vi "Drive and Climb SS Outputs 2017.vi"(11 "Drive Actuator In":T3) -> (0 "error out":T1)   [LabVIEW 2016]
uses:
  Drive Actuator Out 2017.ctl
  Drive and Climb Errors.ctl
  <vilib>/Rock Robotics/WPI/DriverStation/WPI_DriverStationRobotMode2.ctl
  Drive and Climb Logging Values.vi
  Global Variables/Refnum Names.vi
  <vilib>/Rock Robotics/WPI/Solenoid/WPI_SolenoidSetEnum.vi
  Global Variables/Robot Status.vi
  Robot Global Data.vi
  Global Variables/Sensor Data.vi
panel:
  out "Right Drive Commanded Speed":dbl
  out "Right Sensor Velocity":dbl
  out "Left Drive Commanded Speed":dbl
  out "Left Sensor Velocity":dbl
  out "Right Drive Motors":T2(graph)
  out "Left Drive Motors":T2(graph)
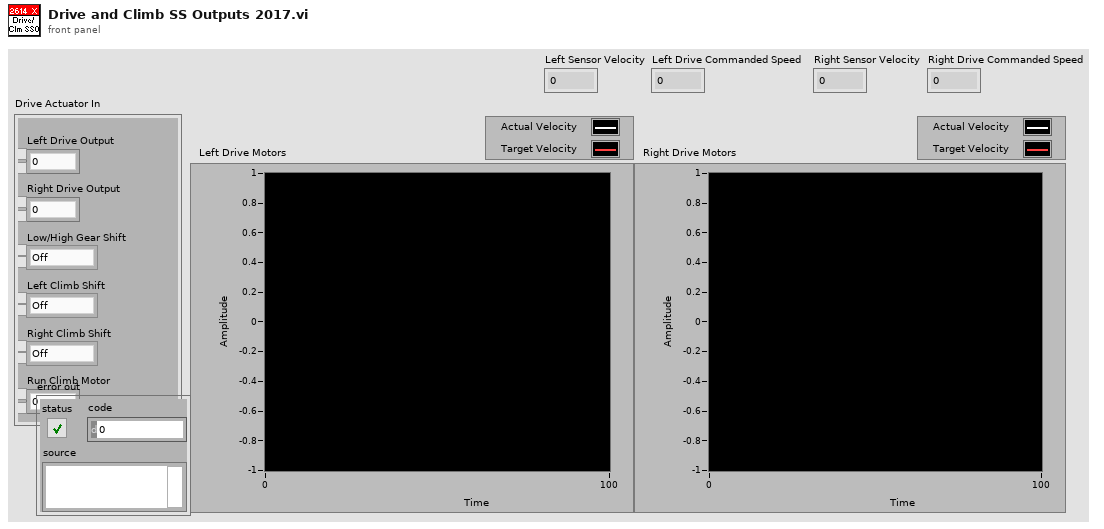
[diagram p1: front panel]
types:
  T1 = typedef "Drive and Climb Errors.ctl" = errorcluster
  T2 = cluster{"Encoder Velocity":dbl, "Left Drive Output":dbl}
  T3 = typedef "Drive Actuator Out 2017.ctl" = cluster{"Left Drive Output":dbl, "Right Drive Output":dbl, "Low/High Gear Shift":enum16{"Off", "On", "Forward", "Reverse"}, "Left Climb Shift":enum16{"Off", "On", "Forward", "Reverse"}, "Right Climb Shift":enum16{"Off", "On", "Forward", "Reverse"}, "Run Climb Motor":dbl}
  T4 = typedef "WPI_DriverStationRobotMode2.ctl" = enum16{"Autonomous Disabled", "Autonomous Enabled", "Teleop Disabled", "Teleop Enabled", "Disconnected", "Finish", "Test Disabled", "Test Enabled", "Emergency Stopped"}
  T5 = typedef "WPI_SolenoidDevRef.ctl" = cluster{"DevStatus":errorcluster, "Pneumatics Control Module":u8, "Forward Solenoid Channel":T6, "Reverse Solenoid Channel":T6}
  T6 = typedef "WPI_SolenoidChannel.ctl" = enum8{"Solenoid 0", "Solenoid 1", "Solenoid 2", "Solenoid 3", "Solenoid 4", "Solenoid 5", "Solenoid 6", "Solenoid 7", "Invalid"}
  T7 = typedef "WPI_MotorControlDeviceRef.ctl" = cluster{"DeviceStatus":errorcluster, "Type":T8, "PWM":cluster{"PWM Channel":T9, "DeadBand":T10}, "CAN":cluster{"Device Number":u8, "SetOutput VI Ref":variant, "GetOutput VI Ref":variant, "Enable VI Ref":variant, "Disable VI Ref":variant, "Data":variant}, "Invert":bool}
  T8 = typedef "WPI_MotorControlType.ctl" = enum16{"PWM", "CAN"}
  T9 = typedef "FPGA_DIOPWMChannel.ctl" = enum8{"PWM 0", "PWM 1", "PWM 2", "PWM 3", "PWM 4", "PWM 5", "PWM 6", "PWM 7", "PWM 8", "PWM 9", "PWM MXP 0", "PWM MXP 1", "PWM MXP 2", "PWM MXP 3", "PWM MXP 4", "PWM MXP 5", "PWM MXP 6", "PWM MXP 7", "PWM MXP 8", "PWM MXP 9", "Invalid"}
  T10 = typedef "WPI_PWMDeadband.ctl" = cluster{"Name":string, "maxPositivePwm":i32, "minPositivePwm":i32, "centerPwm":i32, "maxNegativePwm":i32, "minNegativePwm":i32, "angularRange":u16}
  T11 = typedef "WPI_CANTalonSRX_GlobalStatus.ctl" = cluster{"Applied Throttle":dbl, "Module Enabled":bool, "CAN Error":errorcluster, "Closed Loop Error":dbl, "Forward Limit Switch Closed":bool, "Reverse Limit Switch Closed":bool, "Sensor Position":dbl, "Sensor Velocity":dbl, "Current":dbl, "Sticky Fault - Over Temp":bool, "Sticky Fault - Under Voltage":bool, "Sticky Fault - Forward Limit":bool, "Sticky Fault - Reverse Limit":bool, "Sticky Fault - Forward Soft Limit":bool, "Sticky Fault - Reverse Soft Limit":bool, "Brake is Enabled":bool, "Encoder Position":dbl, "Encoder Velocity":dbl, "Encoder Index Count":dbl, "Encoder A Pin State":bool, "Encoder B Pin State":bool, "Encoder Index Pin State":bool, "Analog In":dbl, "Analog In Velocity":dbl, "Temperature (C)":dbl, "Battery Voltage":dbl, "Control 5 Is Supported":bool, "Current Profile Slot Select":dbl, "Pos Div 8":bool, "Vel Div 4":bool, "Pulse Width Position":i32, "Pulse Width Velocity":i32, "Pulse Width Rise To Rise (us)":i32, "Pulse Width Rise To Fall (us)":i32, "Mot Prof Active Is Under Run":bool, "Mot Prof Active Has Under Run":bool, "Mot Prof Active Is Last":bool, "Mot Prof Active Velocity Only":bool, "Mot Prof Active Is Valid":bool, "Mot Prof Buffer Is Full":bool, "Mot Prof Active Profile Slot Select":i32, "Mot Prof NextID":i32, "Mot Prof Count":i32, "Mot Prof Active Velocity":dbl, "Mot Prof Active Position":dbl, "Mot Prof Output Enable":i32, "UsageFrame":u32, "Motion Magic Active Trajectory":cluster{"Velocity":dbl, "Position":dbl}}
  T12 = cluster{"Sensor Velocity":dbl, "Right Drive Output":dbl}
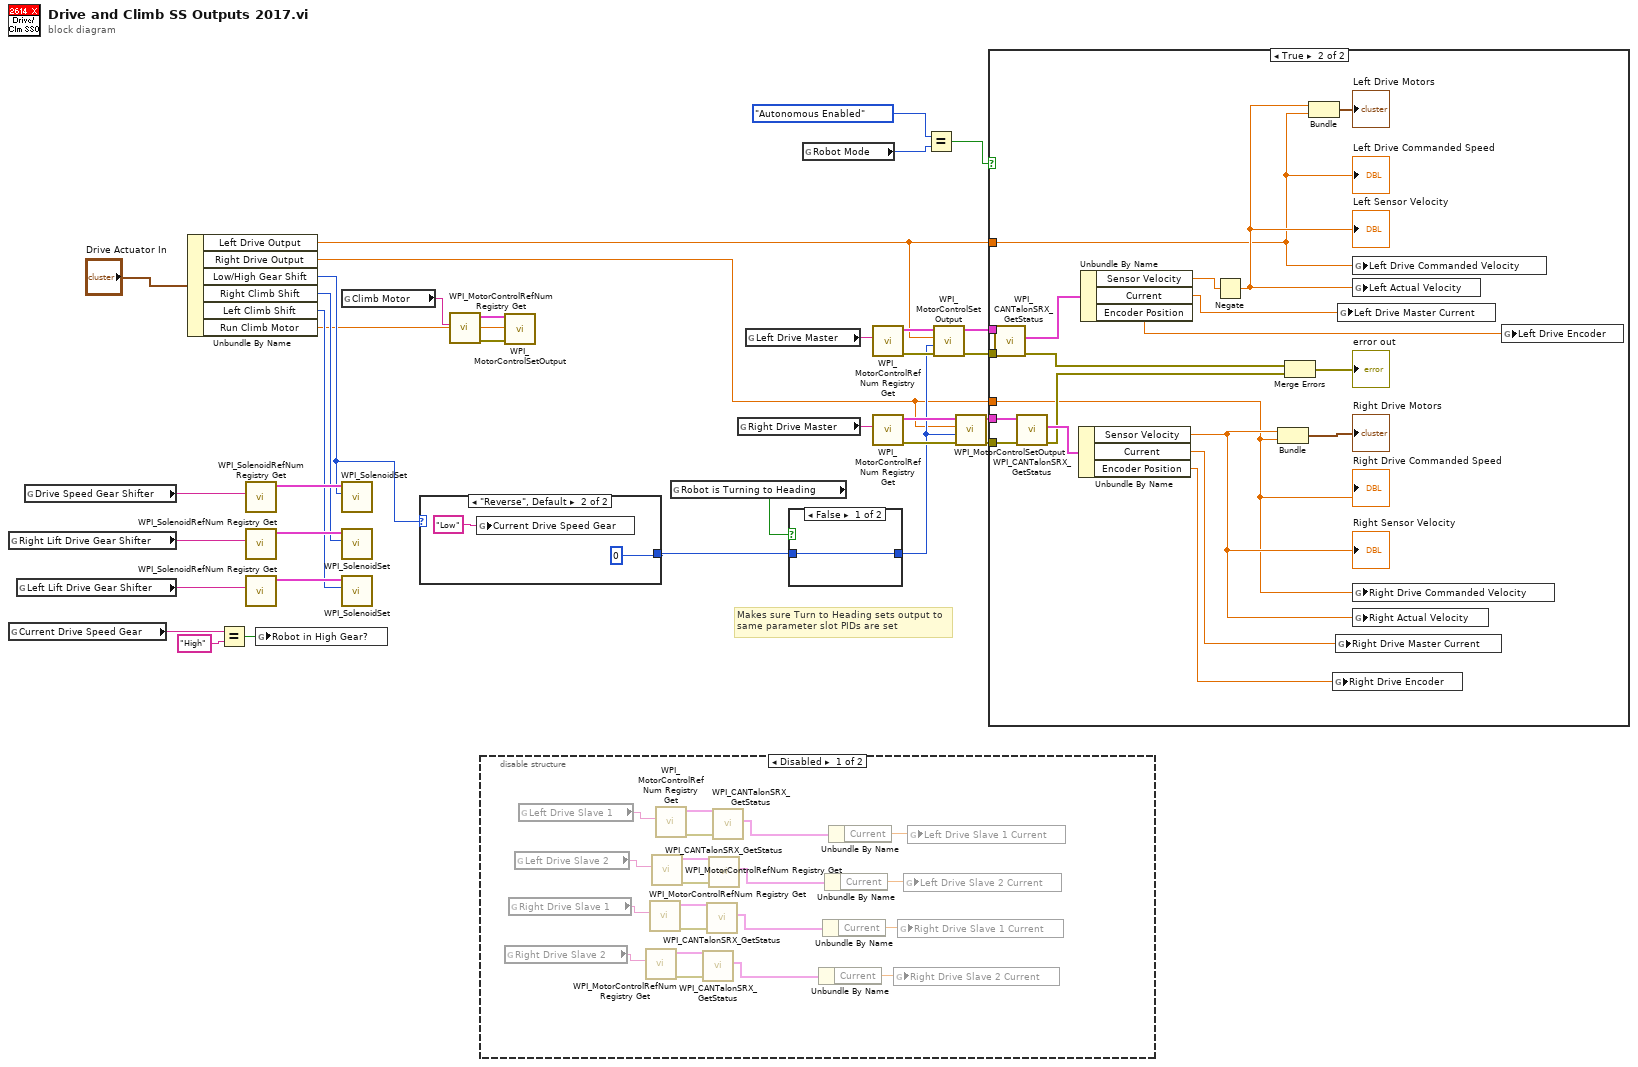
[diagram p0: block diagram]
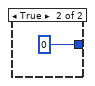
[diagram p4: hidden frame]
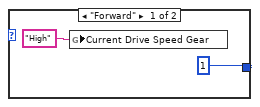
[diagram p5: hidden frame]
diagram:
  # "Makes sure Turn to Heading sets output to same parameter slot PIDs are set"
  n1 = global read "Refnum Names.vi" "Right Lift Drive Gear Shifter"() -> (w22:string)
  n2 = global read "Drive and Climb Logging Values.vi" "Current Drive Speed Gear"() -> (w12:string)
  n3 = global read "Refnum Names.vi" "Left Lift Drive Gear Shifter"() -> (w19:string)
  n4 = global read "Refnum Names.vi" "Drive Speed Gear Shifter"() -> (w30:string)
  n5 = Unbundle By Name("Drive Actuator In") -> ("Left Drive Output"=w8:dbl, "Right Drive Output"=w9:dbl, "Low/High Gear Shift"=w10:enum16{"Off", "On", "Forward", "Reverse"}, "Right Climb Shift"=w17:enum16{"Off", "On", "Forward", "Reverse"}, "Left Climb Shift"=w16:enum16{"Off", "On", "Forward", "Reverse"}, "Run Climb Motor"=w4:dbl)
  n6 = Equal?(x=w12, y="High") -> (x = y?=w15:bool)
  n7 = call <vilib>:"WPI_SolenoidRefNum Registry Get.vi"("refnum name"=w30) -> ("SolenoidDevRef"=w29:T5)  [unwired: 9 in, 1 out]
  n8 = call <vilib>:"WPI_SolenoidRefNum Registry Get.vi"("refnum name"=w22) -> ("SolenoidDevRef"=w21:T5)  [unwired: 9 in, 1 out]
  n9 = call <vilib>:"WPI_SolenoidRefNum Registry Get.vi"("refnum name"=w19) -> ("SolenoidDevRef"=w20:T5)  [unwired: 9 in, 1 out]
  n10 = global write "Robot Status.vi" "Robot in High Gear?"(w15) -> ()
  n11 = global read "Refnum Names.vi" "Climb Motor"() -> (w7:string)
  n12 = call-poly <vilib>:"WPI_SolenoidSet.vi"("Value"=w10, "SolenoidDevRef"=w29) -> ()  [unwired: 8 in, 2 out]
  n13 = call-poly <vilib>:"WPI_SolenoidSet.vi"("Value"=w17, "SolenoidDevRef"=w21) -> ()  [unwired: 8 in, 2 out]
  n14 = call-poly <vilib>:"WPI_SolenoidSet.vi"("Value"=w16, "SolenoidDevRef"=w20) -> ()  [unwired: 8 in, 2 out]
  n15 = case shown="\"Reverse\", Default" w10 {
    tunnel: [u8 1 ("options") u8 0 ("options")] -> w11
    frame "Forward" {
      n16 = global write "Drive and Climb Logging Values.vi" "Current Drive Speed Gear"("High") -> ()
    }
    frame "Reverse", Default {
      n17 = global write "Drive and Climb Logging Values.vi" "Current Drive Speed Gear"("Low") -> ()
    }
  }
  n18 = call <vilib>:"WPI_MotorControlRefNum Registry Get.vi"("refnum name"=w7) -> ("error out"=w6:errorcluster, "MotorControlDevRef"=w5:T7)  [unwired: 9 in]
  n19 = disable-structure shown="Disabled" {
    frame Disabled {
      n20 = global read "Refnum Names.vi" "Right Drive Slave 2"() -> (w44:string)
      n21 = global read "Refnum Names.vi" "Right Drive Slave 1"() -> (w49:string)
      n22 = global read "Refnum Names.vi" "Left Drive Slave 2"() -> (w54:string)
      n23 = global read "Refnum Names.vi" "Left Drive Slave 1"() -> (w59:string)
      n24 = call <vilib>:"WPI_MotorControlRefNum Registry Get.vi"("refnum name"=w44) -> ("error out"=w42:errorcluster, "MotorControlDevRef"=w43:T7)  [unwired: 9 in]
      n25 = call <vilib>:"WPI_MotorControlRefNum Registry Get.vi"("refnum name"=w49) -> ("error out"=w47:errorcluster, "MotorControlDevRef"=w48:T7)  [unwired: 9 in]
      n26 = call <vilib>:"WPI_MotorControlRefNum Registry Get.vi"("refnum name"=w54) -> ("error out"=w52:errorcluster, "MotorControlDevRef"=w53:T7)  [unwired: 9 in]
      n27 = call <vilib>:"WPI_MotorControlRefNum Registry Get.vi"("refnum name"=w59) -> ("error out"=w57:errorcluster, "MotorControlDevRef"=w58:T7)  [unwired: 9 in]
      n28 = call <vilib>:"WPI_CANTalonSRX_GetStatus.vi"("error in (no error)"=w42, "CAN Talon SRX Ref"=w43) -> ("Talon SRX Status"=w41:T11)  [unwired: 7 in, 2 out]
      n29 = call <vilib>:"WPI_CANTalonSRX_GetStatus.vi"("error in (no error)"=w47, "CAN Talon SRX Ref"=w48) -> ("Talon SRX Status"=w46:T11)  [unwired: 7 in, 2 out]
      n30 = call <vilib>:"WPI_CANTalonSRX_GetStatus.vi"("error in (no error)"=w52, "CAN Talon SRX Ref"=w53) -> ("Talon SRX Status"=w51:T11)  [unwired: 7 in, 2 out]
      n31 = call <vilib>:"WPI_CANTalonSRX_GetStatus.vi"("error in (no error)"=w57, "CAN Talon SRX Ref"=w58) -> ("Talon SRX Status"=w56:T11)  [unwired: 7 in, 2 out]
      n32 = Unbundle By Name(w41) -> ("Current"=w40:dbl)
      n33 = Unbundle By Name(w46) -> ("Current"=w45:dbl)
      n34 = Unbundle By Name(w51) -> ("Current"=w50:dbl)
      n35 = Unbundle By Name(w56) -> ("Current"=w55:dbl)
      n36 = global write "Drive and Climb Logging Values.vi" "Right Drive Slave 2 Current"(w40) -> ()
      n37 = global write "Drive and Climb Logging Values.vi" "Right Drive Slave 1 Current"(w45) -> ()
      n38 = global write "Drive and Climb Logging Values.vi" "Left Drive Slave 2 Current"(w50) -> ()
      n39 = global write "Drive and Climb Logging Values.vi" "Left Drive Slave 1 Current"(w55) -> ()
    }
    frame Enabled {
    }
  }
  n40 = call <vilib>:"WPI_MotorControlSetOutput.vi"("error in (no error)"=w6, "Output"=w4, "MotorControlDevRef"=w5) -> ()  [unwired: 6 in, 3 out]
  n41 = global read "Robot Status.vi" "Robot is Turning to Heading"() -> (w14:bool)
  n42 = global read "Refnum Names.vi" "Right Drive Master"() -> (w31:string)
  n43 = global read "Refnum Names.vi" "Left Drive Master"() -> (w35:string)
  n44 = case shown="False" w14 {
    tunnel: [w60 u8 0 ("options")] -> w13
    tunnel: w11 -> [w60 _]
    frame False {
    }
    frame True {
    }
  }
  n45 = global read "Robot Global Data.vi" "Robot Mode"() -> (w2:T4)
  n46 = call <vilib>:"WPI_MotorControlRefNum Registry Get.vi"("refnum name"=w35) -> ("error out"=w23:errorcluster, "MotorControlDevRef"=w34:T7)  [unwired: 9 in]
  n47 = call <vilib>:"WPI_MotorControlRefNum Registry Get.vi"("refnum name"=w31) -> ("error out"=w24:errorcluster, "MotorControlDevRef"=w32:T7)  [unwired: 9 in]
  n48 = Equal?(x=WPI_DriverStationRobotMode2."Autonomous Enabled", y=w2) -> (x = y?=w1:bool)
  n49 = call <vilib>:"WPI_MotorControlSetOutput.vi"("error in (no error)"=w23, "options"=w13, "Output"=w8, "MotorControlDevRef"=w34) -> ("error out"=w26:errorcluster, "MotorControlDevRef"=w28:T7)  [unwired: 5 in, 1 out]
  n50 = call <vilib>:"WPI_MotorControlSetOutput.vi"("error in (no error)"=w24, "options"=w13, "Output"=w9, "MotorControlDevRef"=w32) -> ("error out"=w25:errorcluster, "MotorControlDevRef"=w27:T7)  [unwired: 5 in, 1 out]
  n51 = case shown="True" w1 {
    tunnel: w28 -> [_ w76]
    tunnel: w27 -> [_ w75]
    tunnel: w26 -> [_ w74]
    tunnel: w25 -> [_ w73]
    tunnel: w9 -> [_ w67]
    tunnel: w8 -> [_ w66]
    frame False {
    }
    frame True {
      n52 = call <vilib>:"WPI_CANTalonSRX_GetStatus.vi"("error in (no error)"=w74, "CAN Talon SRX Ref"=w76) -> ("error out"=w71:errorcluster, "Talon SRX Status"=w80:T11)  [unwired: 7 in, 1 out]
      n53 = call <vilib>:"WPI_CANTalonSRX_GetStatus.vi"("error in (no error)"=w73, "CAN Talon SRX Ref"=w75) -> ("error out"=w72:errorcluster, "Talon SRX Status"=w81:T11)  [unwired: 7 in, 1 out]
      n54 = Unbundle By Name(w81) -> ("Sensor Velocity"=w68:dbl, "Current"=w64:dbl, "Encoder Position"=w62:dbl)
      "Right Sensor Velocity" <- w68
      n55 = Unbundle By Name(w80) -> ("Sensor Velocity"=w79:dbl, "Current"=w65:dbl, "Encoder Position"=w63:dbl)
      n56 = Negate(x=w79) -> (-x=w69:dbl)
      "Left Sensor Velocity" <- w69
      n57 = Bundle("Sensor Velocity"=w68, "Right Drive Output"=w67) -> (→"Right Drive Motors":T12)  [unwired: 1 in]
      n58 = Merge Errors(w71, w72) -> (→"error out":errorcluster)
      n59 = Bundle(w69, "Left Drive Output"=w66) -> (→"Left Drive Motors":cluster{dbl, "Left Drive Output":dbl})  [unwired: 1 in]
      n60 = global write "Sensor Data.vi" "Right Drive Encoder"(w62) -> ()
      n61 = global write "Drive and Climb Logging Values.vi" "Right Drive Master Current"(w64) -> ()
      n62 = global write "Drive and Climb Logging Values.vi" "Left Drive Master Current"(w65) -> ()
      n63 = global write "Drive and Climb Logging Values.vi" "Left Drive Commanded Velocity"(w66) -> ()
      n64 = global write "Drive and Climb Logging Values.vi" "Left Actual Velocity"(w69) -> ()
      n65 = global write "Drive and Climb Logging Values.vi" "Right Drive Commanded Velocity"(w67) -> ()
      n66 = global write "Drive and Climb Logging Values.vi" "Right Actual Velocity"(w68) -> ()
      n67 = global write "Sensor Data.vi" "Left Drive Encoder"(w63) -> ()
      "Left Drive Commanded Speed" <- w66
      "Right Drive Commanded Speed" <- w67
    }
  }
